vi "write all DO's.vi"(8 "error in (no error)":errorcluster, 10 "Outputs":bool[](array[boolean]), 11 "USB DAQ in":refnum<class "USB DAQ.lvclass">) -> (0 "error out":errorcluster, 3 "USB DAQ out":refnum<class "USB DAQ.lvclass">)   [LabVIEW 2025, in "USB DAQ.lvclass"]
uses:
  USB DAQ.lvclass
  USB DAQ.lvclass/USB DAQ.ctl
  <vilib>/DAQmx/write.llb/DAQmx Write (Digital 1D Bool NChan 1Samp 1Line).vi
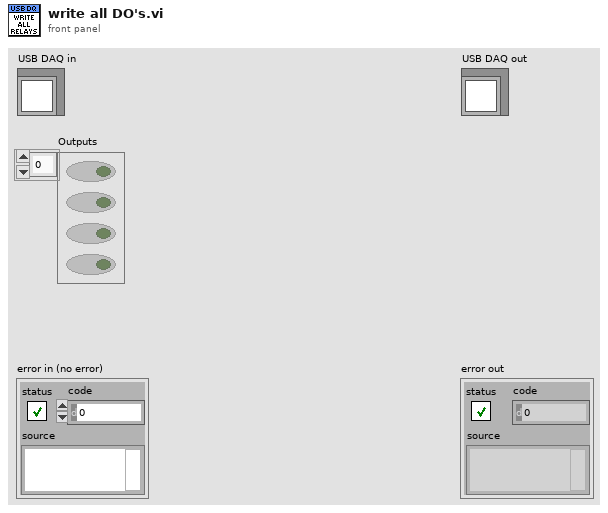
[diagram p1: front panel]
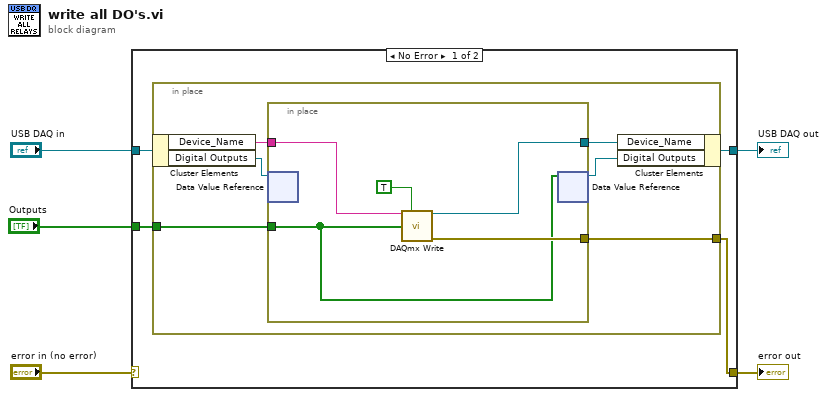
[diagram p0: block diagram]
diagram:
  n1 = case shown="No Error" "error in (no error)" {
    selector: "error in (no error)" -> [_ w22]
    tunnel: [w6 w22] -> w4
    tunnel: [w7 w21] -> w2
    tunnel: "USB DAQ in" -> [w8 w21]
    tunnel: "Outputs" -> [w9 _]
    frame No Error {
      n2 = in-place {
        in-place-border: w9 -> [w15]
        in-place-border: [w12] -> w6
        n3 = in-place-cluster #1(w8) -> ("Device_Name"=w14:string, "Digital Outputs"=w11:refnum<data-value>)
        n4 = in-place {
          in-place-border: w15 -> [w16]
          in-place-border: w14 -> [w20]
          in-place-border: [w18] -> w13
          in-place-border: [w17] -> w12
          n5 = in-place-dvr #2(w11) -> ()  [unwired: 2 out]
          n6 = call-poly <vilib>:"DAQmx Write.vi"("task/channels in"=w20, "auto start"=TRUE, "data"=w16) -> ("task out"=w18:refnum<k21>, "error out"=w17:errorcluster)  [unwired: 10 in, 1 out]
          n7 = in-place-dvr #2(w16) -> (w10:refnum<data-value>)  [unwired: 1 out]
        }
        n8 = in-place-cluster #1("Device_Name"=w13, "Digital Outputs"=w10) -> (w7:refnum<class "USB DAQ.lvclass">)
      }
    }
    frame Error {
    }
  }
  "error out" <- w4
  "USB DAQ out" <- w2
